vi "MesaurementToIdleState.vi"(8 "error in (no error)":errorcluster) -> (0 "error out":errorcluster)   [LabVIEW 2013]
uses:
  Variables/GlobalGetMesaurementStatus.vi
  Variables/StartStopMesaurement.vi
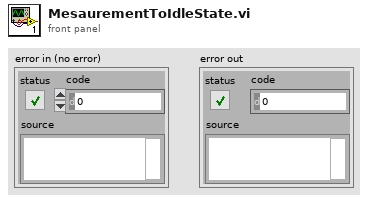
[diagram p1: front panel]
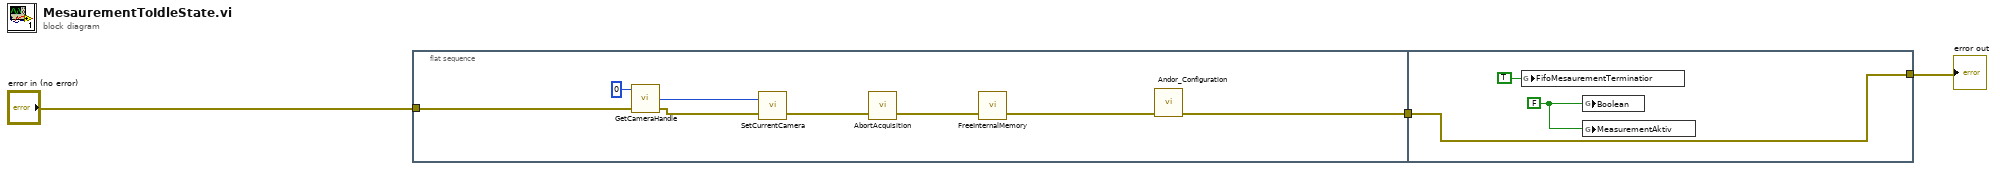
[diagram p0: block diagram]
diagram:
  n1 = flat-sequence {
    tunnel: "error in (no error)" -> [w5]
    tunnel: [w11] -> w3
    tunnel: [w14] -> w1
    tunnel: w3 -> [w14]
    frame #0 {
      n2 = call "GetCameraHandle.vi"("error in (no error)"=w5, "cameraIndex"=0) -> ("error out"=w7:errorcluster, "cameraHandle"=w6:i32)  [unwired: 1 in, 1 out]
      n3 = call "SetCurrentCamera.vi"("error in (no error)"=w7, "cameraHandle"=w6) -> ("error out"=w10:errorcluster)  [unwired: 1 out]
      n4 = call "AbortAcquisition.vi"("error in (no error)"=w10) -> ("error out"=w9:errorcluster)  [unwired: 1 in, 1 out]
      n5 = call "FreeInternalMemory.vi"("error in (no error)"=w9) -> ("error out"=w4:errorcluster)  [unwired: 1 in, 1 out]
      n6 = call "Andor_Configuration.vi"("Error in"=w4) -> ("error out"=w11:errorcluster)  [unwired: 9 in, 1 out]
    }
    frame #1 {
      w12 = FALSE ("Boolean")
      n7 = global write "GlobalGetMesaurementStatus.vi" "FifoMesaurementTerminatior"(TRUE ("FifoMesaurementTerminatior")) -> ()
      n8 = global write "StartStopMesaurement.vi" "Boolean"(w12) -> ()
      n9 = global write "GlobalGetMesaurementStatus.vi" "MeasurementAktiv"(w12) -> ()
    }
  }
  "error out" <- w1
